vi "stop.vi"(3 "error in (no error)":errorcluster, 4 "Device Number":i32=1, 5 "VISA resource name":refnum<visa-resource-name>) -> (0 "error out":errorcluster, 2 "VISA resource name out":refnum<visa-resource-name>)   [LabVIEW 2020]
uses:
  Request.ctl
  ZaberTSeries.lvlib
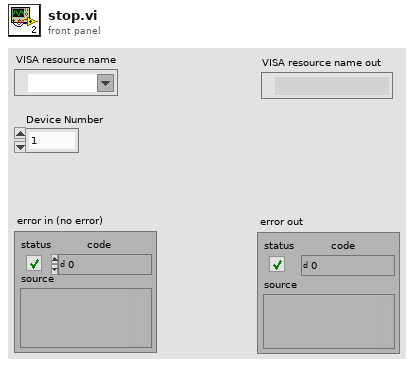
[diagram p1: front panel]
types:
  T1 = typedef "ZaberTSeries.lvlib/Request.ctl" = cluster{"Device Number":u8, "Command":u8, "Data":i32, "Response Count":i32}
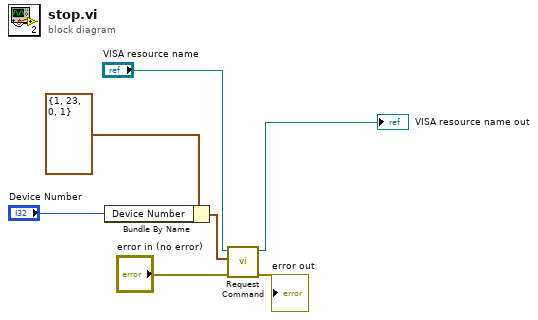
[diagram p0: block diagram]
diagram:
  n1 = Bundle By Name(cluster=T1 {"Device Number"=1, "Command"=23, "Data"=0, "Response Count"=1} ("Request"), "Device Number"="Device Number") -> (w6:T1)
  n2 = call "Request Command.vi"("error in (no error)"="error in (no error)", "Request"=w6, "VISA resource name"="VISA resource name") -> ("error out"=→"error out":errorcluster, "VISA resource name out"=→"VISA resource name out":refnum<visa-resource-name>)  [unwired: 5 in, 2 out]
